vi "數位積分適應性控制_輸入權重係數_隔振(實際控制).vi"() -> ()   [LabVIEW 2010]
uses:
  <vilib>/DAQmx/read.llb/DAQmx Read (Analog DBL 1Chan 1Samp).vi
  <vilib>/DAQmx/write.llb/DAQmx Write (Analog DBL 1Chan 1Samp).vi
  <vilib>/DAQmx/create/channels.llb/DAQmx Create Channel (AI-Voltage-Basic).vi
  <vilib>/DAQmx/configure/timing.llb/DAQmx Timing (Sample Clock).vi
  <vilib>/DAQmx/create/channels.llb/DAQmx Create Channel (AO-Voltage-Basic).vi
  <vilib>/daqmx/miscellaneous.llb/DAQmx Fill In Error Info.vi
  <vilib>/measure/maspectr.llb/FFT Spectrum (Mag-Phase) for 1 Chan.vi
  <vilib>/measure/NI_MAPro.lvlib
panel:
  in  "DA輸出DC濾除":dbl
  out "積分":dbl(graph)
  in  "I增益":dbl=1.0
  in  "averaging parameters":T1={"averaging mode"=enum."No averaging", "weighting mode"=enum."Exponential", "number of averages"=10} {"number of averages" min=1}
  out "magnitude":cluster{"f0":dbl, "df":dbl, "magnitude":dbl[]} {"magnitude" format="%.2p"; "f0" format="%0.2p"; "df" format="%0.2p"}
  out "Waveform Graph":cluster{"f0":dbl, "df":dbl, "magnitude":dbl[]}(graph)
  in  "DAQ input":tag
  in  "DAQ output":tag
  in  "平均數":i32=1
  in  "ÂoDC«á©ñ¤j":dbl=1.0
  in  "Kp":dbl
  out "當下誤差":dbl=0.1 format="%#_13g"
  out "模擬輸入x(t)":dbl[][](graph)
  out "理想與FIR輸出":dbl[][](graph)
  out "message":string=" INSTRUCTIONS:\r\rNormal Use:  When using subVIs that incorporate the error in/error out (or error I/O) structure, place this handler where you want to inform the user of an error, typically at the end of the I/O data path, as the last action of the program.  If the error in error? is ERROR, the handler creates a message describing the error and its source.  If the type of dialog = 1 (default), the message is displayed to the user, who can only acknowedge it.  If the type = 2, the user can acknowledge the message or abort execution; aborting a program with active I/O is not recommended.  If the type = 0, no message is displayed; this is used to process the error programmatically, and the error out cluster elements are wired to individual terminals for that reason.  \r\rOther Use:\n\r\nlocal testing.  To test the error code of a subVI or function that does not have the error I/O structure, you can wire its error code and a source string to the local error code and error source inputs.  If error in error? indicates no error and error code is not equal to 0, the local code and source are substituted for the error in values, and error? is set TRUE (ERROR)."
  out "誤差":dbl(graph)
  out "while平均運行時間":dbl
  out "收斂time":dbl
  out "各頻率誤差已達標準":bool
  in  "各頻率誤差低於多少亮燈":dbl=0.1 format="%#_13g"
  in  "order":i32=100
  in  "取樣頻率":dbl=1000.0 min=1.0 max=1000.0 step=1.0
  in  "stop":bool
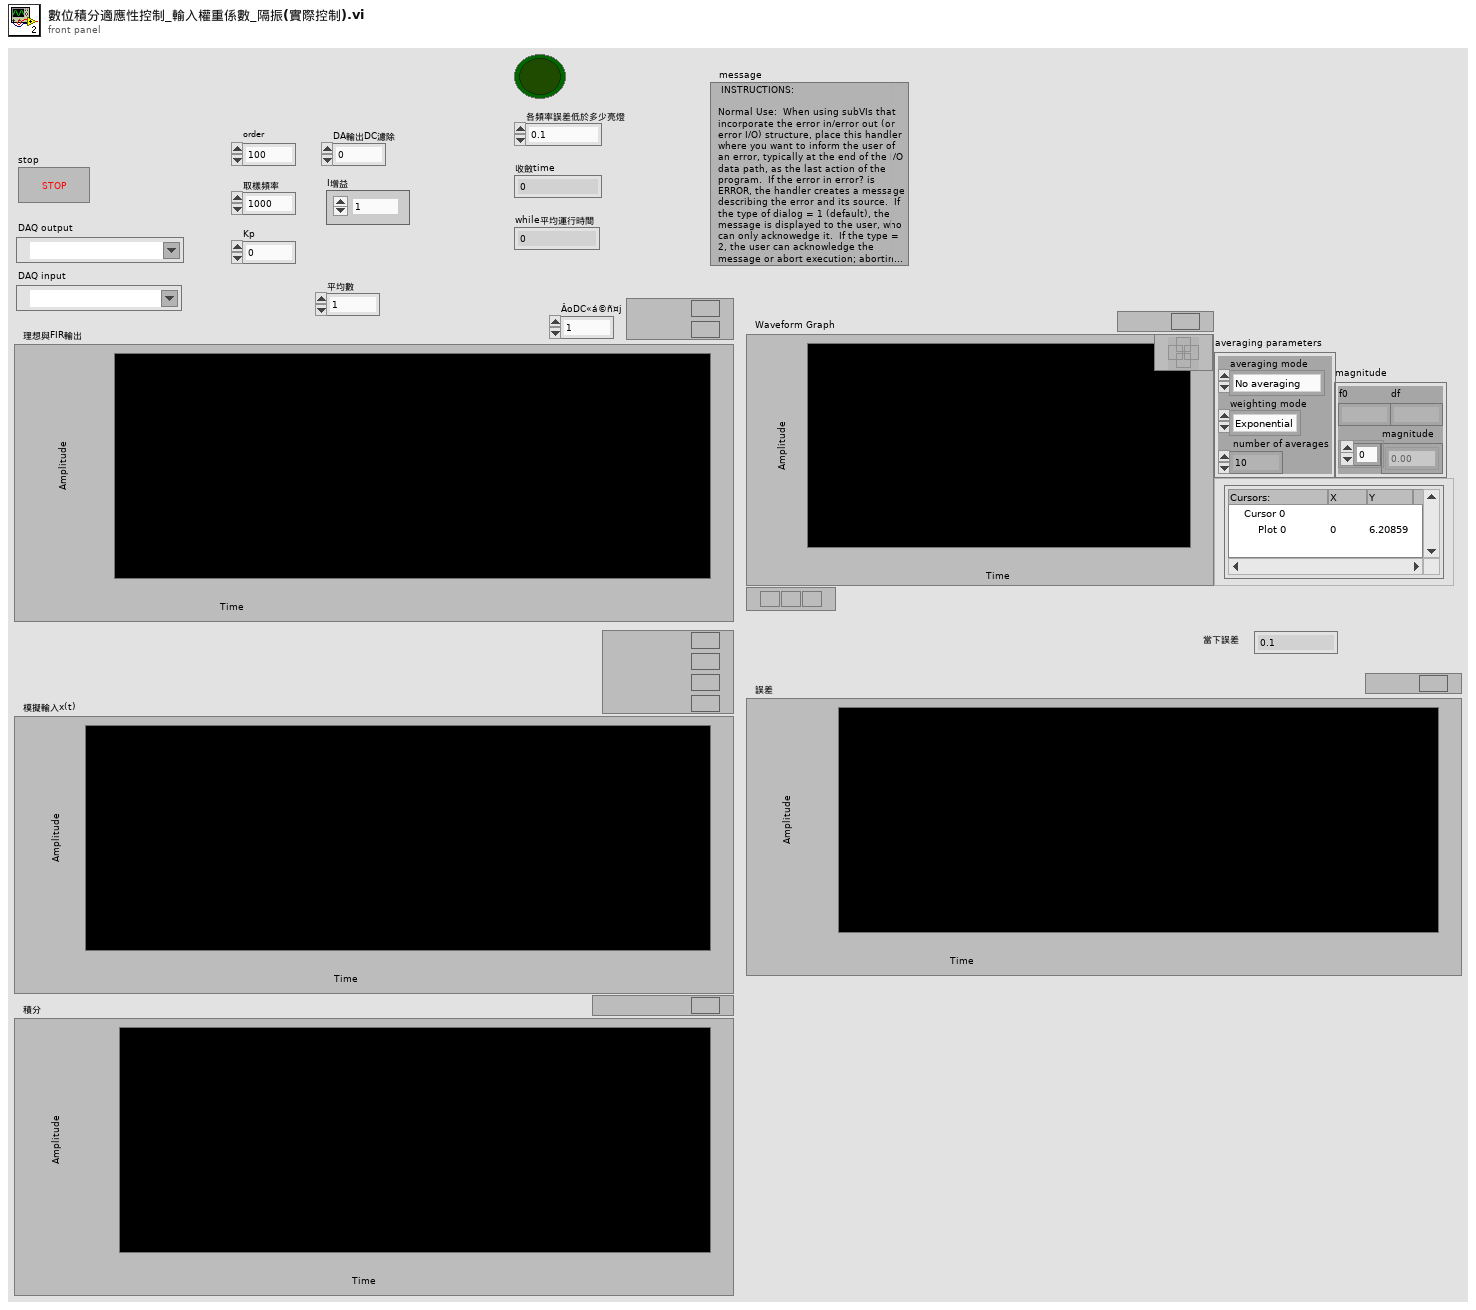
[diagram p1: front panel]
types:
  T1 = cluster{"averaging mode":enum16{"No averaging", "Vector averaging", "RMS averaging", "Peak hold"}, "weighting mode":enum16{"Linear", "Exponential"}, "number of averages":u32}
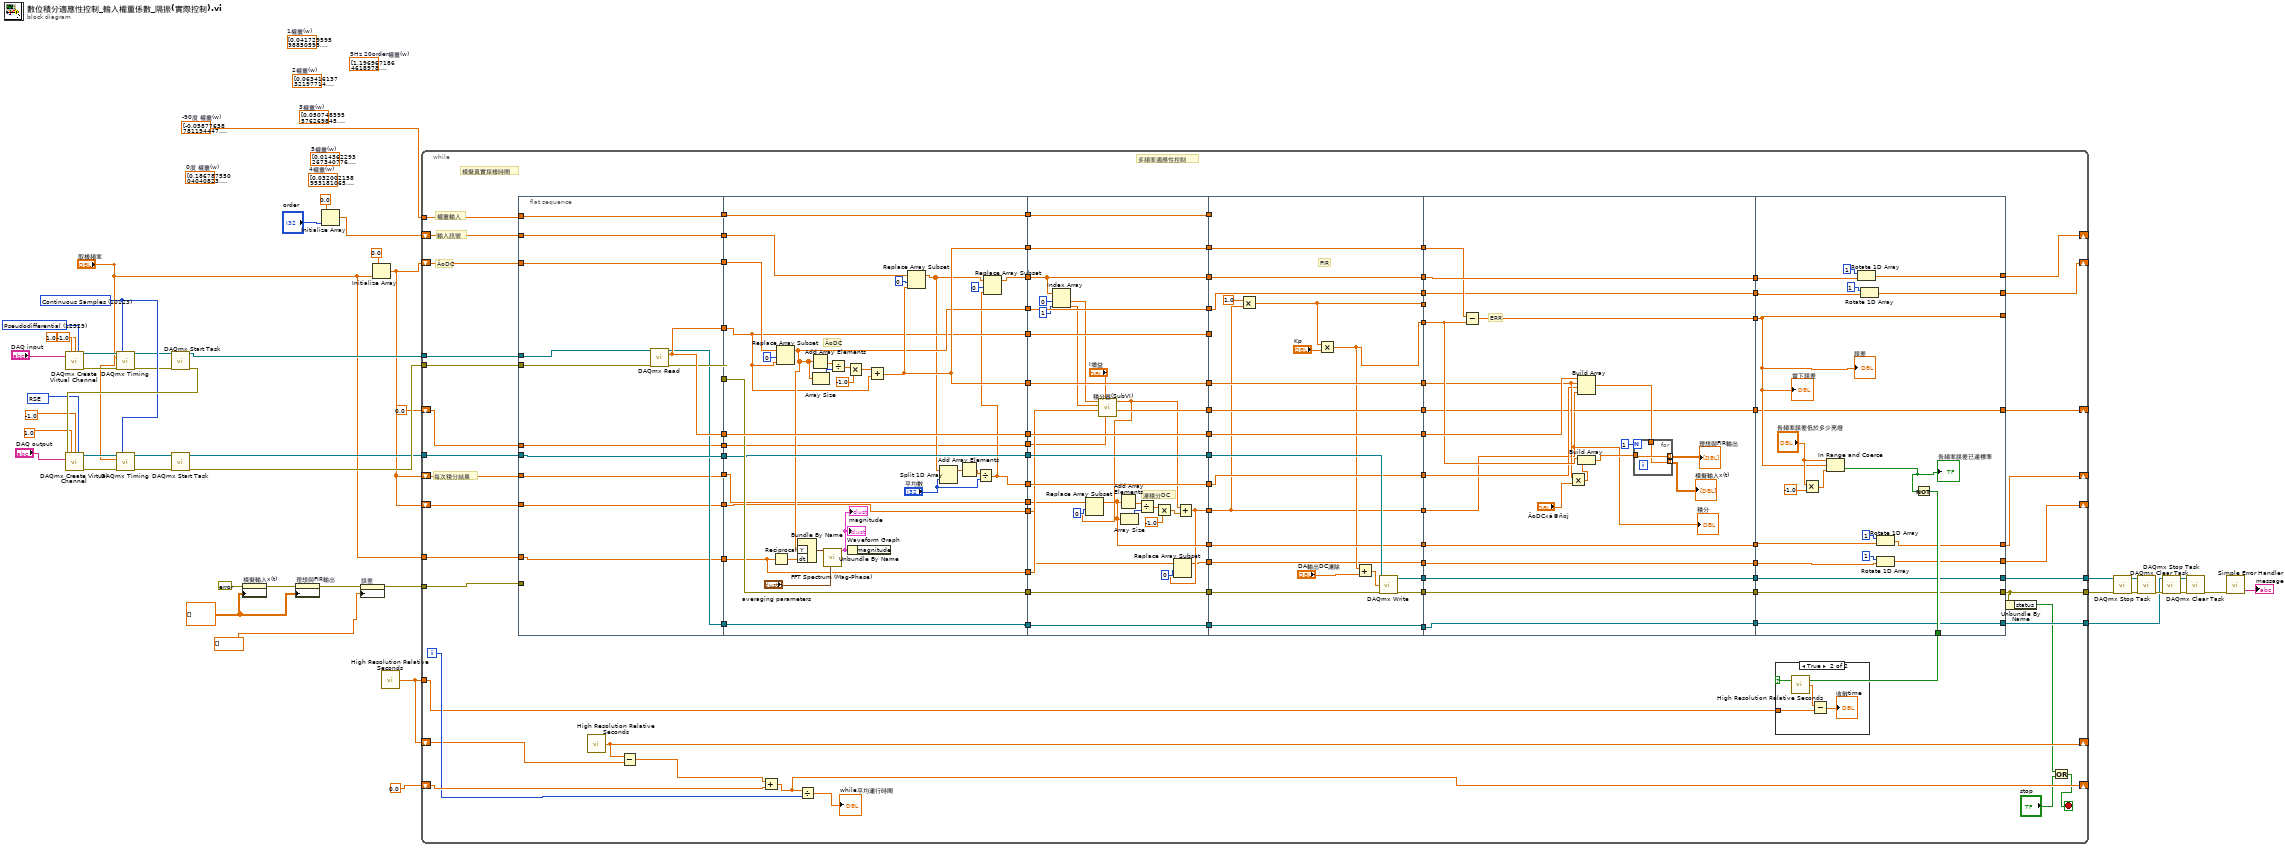
[diagram p0: block diagram]
diagram:
  (unwired) dbl[] [1.1969671864618978, 0.9836479688110593, 0.7683397307293479, 0.5547041148596448, 0.33841914564835257, 0.12405107039492207, -0.09257217575840213, -0.30706835872399124, -0.5236217829176951, -0.7376512261394793, -0.9534881580652202, -1.1673771435073645]  # 5Hz 20order權重(w)
  (unwired) dbl[] [0.04172959598850595, 0.041032000468528444, 0.040333217667049365, 0.03963360238588265, 0.03893205689600781, 0.03822950710044137, 0.03752526162041425, 0.036820019207773794, 0.03611349886737446, 0.03540561191052648, 0.03469552473426457, 0.0339838941268913, 0.03327051237657309, 0.03255595284486474, 0.031839823725201506, 0.03112222992536054, 0.030402869704382152, 0.029681974372377747, 0.02896038916329569, 0.02823777554389203, 0.027514172218931345, 0.026789142915512532, 0.026062835909340894, 0.025335140782112305, 0.0246063929857642, 0.0238764912383573, 0.023144908178161352, 0.022411287738477562, 0.021676068818243868, 0.020939160662649045, 0.020201152434326186, 0.019461448759074126, 0.018720614589735427, 0.017977930182099557, 0.017234725633515236, 0.016490584286721673, 0.01574616922561371, 0.015000724778555387, 0.014255051294173798, 0.013507854465542396, 0.012760442794157674, 0.01201235390633865, 0.011264924754863731, 0.010516019014728371, 0.009767013836059027, 0.009016973363734176, 0.008267381865193765, 0.007517321284663236, 0.006767505174674699, 0.006017229643389848, 0.005267192614920231, 0.004517461974244641, 0.003768561212744832, 0.0030200228117672986, 0.0022719427566014736, 0.0015237938881411776, 0.000776028895793179, 2.8406698505853e-05, -0.0007189560856639669, -0.001466289375680223, -0.0022141752119242833, -0.00296223837493176, -0.0037105231609250904, -0.0044587188414679894, -0.005206880706007413, -0.005954925695853661, -0.006703250220456672, -0.007451258574261906, -0.008198646895597017, -0.00894538586732751, -0.009691718602987901, -0.010437630253585128, -0.011183561844381799, -0.011928876798359233, -0.01267392362649141, -0.013418115373255173, -0.014162730174135814, -0.014907011099846127, -0.015651466362883223, -0.016395255132347217]  # 1權重(w)
  (unwired) dbl[] [0.06341613732197714, 0.06217259987768136, 0.06091889839827501, 0.059657027975942634, 0.05838513130060538, 0.057105429036780835, 0.05581630468491692, 0.05451958671274844, 0.05321400052382132, 0.05190095795462464, 0.0505792924357668, 0.04925037382622508, 0.04791324745250905, 0.04656910885733873, 0.04521739323286119, 0.04385903504088003, 0.04249355654291914, 0.04112170973577467, 0.03974339566502147, 0.038359057729198356, 0.036968896626547745, 0.035573135462967795, 0.03417200396401437, 0.032765454453403224, 0.031353955225041454, 0.029937447677999423, 0.028516571076552054, 0.02709070831884093, 0.025660911022225244, 0.02422642146811649, 0.022788545963313027, 0.02134634309175934, 0.019901312467275358, 0.01845212060283792, 0.017000713743516246, 0.015545555821830101, 0.014088891066951667, 0.01262886119459867, 0.011167931860344331, 0.009704011220608925, 0.00823993912579386, 0.006773494080066802, 0.005307599202569423, 0.0038399997075308293, 0.002373301534065933, 0.0009056073754654906, -0.0005608198104424876, -0.0020274908023066064, -0.00349257184291716, -0.00495735756770476, -0.006420298603255164, -0.007882348498007218, -0.009342158197245886, -0.010800492054227515, -0.012256318746365426, -0.013710262151131126, -0.015161545855611632, -0.016610444212633524, -0.018056301789600413, -0.019499278202438776, -0.02093899944369821, -0.0223752878332073, -0.023808034087866817, -0.025236799410333622, -0.02666156671827483, -0.028081824430815434, -0.029497837036270607, -0.030908780471520174, -0.03231490792980266, -0.033715380043063486, -0.035110769547232086, -0.03650002949596311, -0.037884088770354214, -0.039261583529015806, -0.0406335817714926, -0.0419984699060945, -0.04335769969455247, -0.044709340565506045, -0.046054929901912504, -0.04739266586653418]  # 2權重(w)
  (unwired) dbl[] [0.050748595576269845, 0.04976296352033009, 0.04875982009079402, 0.047739876462819145, 0.046703040375167114, 0.045650133074210314, 0.04458114196253071, 0.043496793229900375, 0.04239715058244961, 0.041282877646379335, 0.04015408828621526, 0.0390114226735173, 0.037855066530000724, 0.03668563212746908, 0.035503373306480325, 0.03430887198349752, 0.03310241847891101, 0.03188456159293401, 0.0306556647988646, 0.029416231366791036, 0.028166666899342822, 0.02690742906046231, 0.02563897199169044, 0.024361700257702942, 0.023076128947505922, 0.021782639152128802, 0.020481775548324012, 0.01917386761510714, 0.017859527855722725, 0.01653903984113062, 0.0152130943393199, 0.013881909276752508, 0.012546252987204293, 0.011206249418488282, 0.009862751954706962, 0.008515824389261194, 0.0071664350548475515, 0.005814557083491869, 0.004461193842393036, 0.0031062458409534983, 0.0017508549797988996, 0.00039490673524854455, -0.0009604508081786534, -0.00231532314495768, -0.0036687042224219026, -0.005020621356114889, -0.006370100664414814, -0.007717078846704026, -0.009060706958838661, -0.010400857399114933, -0.011736764664452096, -0.013068202046663332, -0.014394482563247228, -0.015715318779835633, -0.017030103015260322, -0.018338500437555277, -0.019639965699944875, -0.02093411125155473, -0.022220425174011453, -0.023498500316211767, -0.02476788628580389, -0.026028118442952625, -0.027278791828652713, -0.028519397215787497, -0.02974957386421309, -0.030968771963779416, -0.03217669828069134, -0.03337276891488156, -0.03455672003560269, -0.03572794343441583, -0.03688624362071261, -0.03803098771018863, -0.03916204565148949, -0.040278760392357484, -0.04138104888125941, -0.04246819906988395, -0.04354020353707057, -0.044596264993009734, -0.04563644214557537, -0.04666003862461791]  # 3權重(w)
  (unwired) dbl[] [0.032002158953181065, 0.03127382782707821, 0.030526170728283758, 0.029759763274351574, 0.028974940151298634, 0.028172378359730542, 0.027352456089560346, 0.026515818667865988, 0.025662886279247437, 0.024794305076083024, 0.023910519758936682, 0.02301218583560877, 0.02209978347650994, 0.021173970069008865, 0.020235260678732485, 0.019284323422338375, 0.018321690205268765, 0.017348029489250138, 0.016363905805265377, 0.015369992436563043, 0.014366868017920408, 0.013355206162749383, 0.012335601950499554, 0.011308724669250866, 0.010275192231125899, 0.009235674439598471, 0.008190803514180603, 0.007141236482790735, 0.0060876291688448, 0.005030624411114561, 0.003970920999492173, 0.00290914229363768, 0.0018460084806794317, 0.0007821062594628047, -0.0002817977090353781, -0.0013451554114184553, -0.0024071324122346663, -0.0034672373752764407, -0.004524596908236169, -0.005578769187484147, -0.006628807944435608, -0.007674293764050601, -0.00871429127788735, -0.009748368669830114, -0.010775668901956829, -0.01179573002527658, -0.01280774449609574, -0.013811208806555973, -0.014805384765904395, -0.015789748218182048, -0.016763619606387455, -0.017726453762181474, -0.018677602391468765, -0.019616511384402242, -0.02054258465159873, -0.021455266160387752, -0.022353998874567755, -0.023238226548113566, -0.02410741351803644, -0.024961012340757562, -0.02579852094447031, -0.026619400014715532, -0.02742317752943987, -0.02820932418227676, -0.02897739076641073, -0.029726858427100978, -0.030457326187173502, -0.031168284206444605, -0.031859363152719686, -0.03253006838100269, -0.033180076868829615, -0.03380889649251497, -0.034416256941201144, -0.035001681449908936, -0.035564938807506684, -0.03610554595895217, -0.0366233294436314, -0.037117764767889326, -0.037588745519972454, -0.038035863428471775]  # 4權重(w)
  (unwired) dbl[] [0.014362293267340776, 0.013689395410719023, 0.01300309315294107, 0.012304038900019095, 0.011592878877058704, 0.010870379633601756, 0.010137194353703931, 0.009394105249200462, 0.00864177649435847, 0.00788101488995614, 0.007112496730501849, 0.006337046071486811, 0.005555358538019961, 0.004768287479898683, 0.003976539913125064, 0.003180982341088728, 0.002382325980315668, 0.0015814283651622496, 0.0007790146642582781, -2.4054313914244825e-05, -0.000827057668575488, -0.0016291403226613053, -0.0024295741343070406, -0.0032275334039682992, -0.004022269261344749, -0.0048129686579806655, -0.00559888187871097, -0.006379225608899076, -0.007153234872105012, -0.007920156980446848, -0.008679209089775429, -0.009429667974273952, -0.010170745252987659, -0.010901778533758563, -0.011621962330653905, -0.012330695089693547, -0.013027139313185958, -0.013710766073403635, -0.014380735105048734, -0.015036588270713053, -0.015677454578137223, -0.016302915317597706, -0.016912126659931886, -0.0175047023962845, -0.018079862708683603, -0.018637231671910448, -0.01917608031986532, -0.01969603812834782, -0.02019644130835423, -0.020676932921196416, -0.021136920452136273, -0.021576054554505567, -0.02199380752971395, -0.022389849161288427, -0.0227637296729414, -0.023115144960455324, -0.023443713070951836, -0.02374914535548648, -0.024031129622389645, -0.024289402699926976, -0.024523719881827128, -0.024733831852911652, -0.024919569057548743, -0.02508070675145801, -0.0252171314190388, -0.02532864160374426, -0.025415208320913384, -0.0254766588913466, -0.025513034867214377, -0.02552418292972814, -0.02551021895948809, -0.025471025546434167, -0.025406810325759623, -0.02531747583831068, -0.025203309274158328, -0.025064224461733845, -0.024900580975780743, -0.02471227517816193, -0.024499764141358703, -0.024263080705131754]  # 5權重(w)
  (unwired) dbl[] [0.18678755004040823, 0.17882619748458314, 0.170712296455689, 0.16245257152505876, 0.15405454867553942, 0.14552523682324905, 0.13687159530574372, 0.12810196462388707, 0.11922362147035999, 0.11024393073088701, 0.10117036364485271, 0.09201149209306575, 0.08277436332911685, 0.07346739409850038, 0.06409841525561331, 0.05467582605915196, 0.04520705780003369, 0.03570079633951639, 0.02616517534237316, 0.016608099867348597, 0.007037550190427917, -0.002537488532805972, -0.012109386514070251, -0.021670078710663815, -0.031211136355664814, -0.04072404103843337, -0.050201506295751895, -0.059634697247062, -0.06901578876295462, -0.07833678686397391, -0.0875896165139027, -0.09676628530049372, -0.1058592127633476, -0.11486053312230449, -0.12376230508663352, -0.13255713450591536, -0.1412373426283469, -0.1497958727547784, -0.15822474190263155, -0.1665175154150831, -0.1746667650614144, -0.18266518234592094, -0.19050584543113128, -0.1981828435843626, -0.2056888768059049, -0.2130178209590218, -0.22016340348000582, -0.22711953829571419, -0.233880164162633, -0.24043951812605066, -0.2467920977101983, -0.25293205077048525, -0.2588545397521522, -0.2645544847915611, -0.27002654535583903, -0.2752661953902621, -0.28026944958627037, -0.28503187047512585, -0.28954881763286344, -0.29381678537090966, -0.29783232335913956, -0.30159129471393037, -0.3050912331475972, -0.30832924646728915, -0.3113020963534453, -0.3140069410480377, -0.31644199138653817, -0.3186047046785827, -0.3204935982376899, -0.32210684992236727, -0.32344335057664403, -0.3245013187862961, -0.3252801022894491, -0.32577926591498596, -0.32599826290987993, -0.32593663650954463, -0.32559487153422917, -0.3249726147434439, -0.3240708551869918, -0.3228901701852509]  # 0度 權重(w)
  w4 = dbl[] [-0.05877658781194447, -0.05880165783072071, -0.058769626713902144, -0.05868052843544654, -0.05853445290663261, -0.05833154600716313, -0.05807200513047942, -0.05775609051408422, -0.05738411490100067, -0.05695643829566999, -0.05647347561480095, -0.05593570222205698, -0.05534364366063041, -0.0546978771243554, -0.05399903471184836, -0.05324779605889828, -0.052444887701321614, -0.05159109221709506, -0.050687246789522196, -0.04973422883689582, -0.04873296289280662, -0.04768442344356334, -0.046589627008202315, -0.04544963505892205, -0.044265561327572645, -0.043038556514139834, -0.041769807581880536, -0.04046054418500069, -0.03911204002747684, -0.03772560321594224, -0.0363025799259075, -0.03484435512137173, -0.033352340191170726, -0.03182797732145333, -0.030272749521124433, -0.02868816831319295, -0.027075769660101768, -0.025437116513894426, -0.02377379954828862, -0.022087426486926968, -0.020379633339138514, -0.018652081796517977, -0.01690644743242602, -0.01514441726000822, -0.013367701416755104, -0.01157802234878765, -0.009777114554821144, -0.007966727150988276, -0.006148619219587733, -0.00432454880331794, -0.0024962812704839394, -0.0006655945165545307, 0.0011657354252903728, 0.002995933356237631, 0.004823221823050019, 0.006645830331619849, 0.00846199503756085, 0.010269953129429738, 0.012067944536500928, 0.01385422736721719, 0.015627071128350007, 0.01738475403707428, 0.01912557209081219, 0.020847837381648134, 0.022549872651853698, 0.02423002464683928, 0.02588666747979125, 0.027518193376758496, 0.029123015099837102, 0.03069957472506095, 0.032246340970037195, 0.03376180823956406, 0.035244507411115795, 0.036693002110996215, 0.038105881963939006, 0.039481769906701984, 0.04081933200018057, 0.042117268135363845, 0.04337431575808651, 0.04458925443984995]  # -90度 權重(w)
  w31 = 10123 items=["Finite Samples"=10178, "Continuous Samples"=10123, "Hardware Timed Single Point"=12522] ("sample mode")
  w28 = 10083 items=["Default"=-1, "RSE"=10083, "Differential"=10106, "Pseudodifferential"=12529] ("output terminal configuration")
  w27 = 12529 items=["default"=-1, "RSE"=10083, "NRSE"=10078, "Differential"=10106, "Pseudodifferential"=12529] ("input terminal configuration")
  w35 = dbl[][] [] ("History Data")
  n1 = call-poly <vilib>:"DAQmx Create Virtual Channel.vi"("maximum value"=1.0, "minimum value"=-1.0, "input terminal configuration"=w27, "physical channels"="DAQ input") -> ("task out"=w19:refnum<k21>, "error out"=w22:errorcluster)  [unwired: 10 in]
  n2 = call-poly <vilib>:"DAQmx Timing.vi"("task/channels in"=w19, "sample mode"=w31, "rate"="取樣頻率", "error in"=w22) -> ("task out"=w20:refnum<k21>, "error out"=w21:errorcluster)  [unwired: 10 in]
  n3 = call <vilib>:"DAQmx Start Task.vi"("task/channels in"=w20, "error in"=w21) -> ("task out"=w18:refnum<k21>, "error out"=w34:errorcluster)  [unwired: 12 in]
  n4 = call-poly <vilib>:"DAQmx Create Virtual Channel.vi"("maximum value"=1.0, "minimum value"=-1.0, "output terminal configuration"=w28, "physical channels"="DAQ output", "error in"=w34) -> ("task out"=w26:refnum<k21>, "error out"=w23:errorcluster)  [unwired: 9 in]
  n5 = call-poly <vilib>:"DAQmx Timing.vi"("task/channels in"=w26, "sample mode"=w31, "rate"="取樣頻率", "error in"=w23) -> ("task out"=w25:refnum<k21>, "error out"=w24:errorcluster)  [unwired: 10 in]
  n6 = call <vilib>:"DAQmx Start Task.vi"("task/channels in"=w25, "error in"=w24) -> ("task out"=w16:refnum<k21>, "error out"=w17:errorcluster)  [unwired: 12 in]
  n7 = property on="模擬輸入x(t)" class="WFChart (strict)"(error in=errorcluster {"status"=FALSE, "code"=0, "source"=""} ("error constant"), "History Data"=w35) -> (error out=w41:errorcluster)  [unwired: 1 in, 1 out]
  n8 = property on="理想與FIR輸出" class="WFChart (strict)"(error in=w41, "History Data"=w35) -> (error out=w42:errorcluster)  [unwired: 1 in, 1 out]
  n9 = Initialize Array(0.0 ("element"), "order") -> (w37:dbl[])
  n10 = property on="誤差" class="WFChart (strict)"(error in=w42, "History Data"=dbl[] []) -> (error out=w44:errorcluster)  [unwired: 1 in, 1 out]
  n11 = Initialize Array(0.0 ("element"), "取樣頻率") -> (w1:dbl[])
  n12 = call <vilib>:"High Resolution Relative Seconds.vi"() -> ("relative seconds"=w46:dbl)
  n13 = while {
    shift-right: [w123] -> _
    shift-left: w37 -> [w143]
    tunnel: w46 -> [w129]
    shift-right: [w130] -> _
    shift-left: w46 -> [w128]
    shift-right: [w131] -> _
    shift-left: 0.0 -> [w133]
    tunnel: w44 -> [w126]
    tunnel: w4 -> [w140]
    shift-right: [w117] -> _
    shift-left: w1 -> [w119]
    tunnel: w18 -> [w113]
    tunnel: w17 -> [w112]
    tunnel: w16 -> [w111]
    tunnel: [w107] -> w10
    tunnel: [w98] -> w9
    tunnel: [w101] -> w8
    tunnel: "取樣頻率" -> [w95]
    shift-right: [w67] -> _
    shift-left: 0.0 ("element") -> [w65]
    shift-right: [w55] -> _
    shift-left: w1 -> [w62]
    shift-right: [w48] -> _
    shift-left: w1 -> [w53]
    i -> [w132]
    stop <- w100 stop-if-true
    # "每次積分結果"
    # "權重輸入"
    # "輸入訊號"
    # "ÂoDC"
    # "模擬真實採樣時間"
    # "多頻率適應性控制"
    n14 = flat-sequence {
      tunnel: [w160] -> w144
      tunnel: w143 -> [w160]
      tunnel: [w155] -> w142
      tunnel: [w159] -> w141
      tunnel: w140 -> [w159]
      tunnel: w126 -> [_]
      tunnel: [w155] -> w124
      tunnel: [w154] -> w122
      tunnel: w119 -> [w158]
      tunnel: [w158] -> w118
      tunnel: w113 -> [w157]
      tunnel: w112 -> [w156]
      tunnel: w111 -> [w153]
      tunnel: [w153] -> w110
      tunnel: [w152] -> w104
      tunnel: w95 -> [w151]
      tunnel: [w151] -> w94
      tunnel: [w150] -> w66
      tunnel: w65 -> [w150]
      tunnel: [w149] -> w63
      tunnel: w62 -> [w149]
      tunnel: [w148] -> w54
      tunnel: w53 -> [w148]
      tunnel: w144 -> [w191]
      tunnel: w142 -> [w169]
      tunnel: [w167] -> w93
      tunnel: [w192] -> w91
      tunnel: w141 -> [w192]
      tunnel: [w188] -> w89
      tunnel: [w190] -> w87
      tunnel: w124 -> [w190]
      tunnel: w122 -> [w188]
      tunnel: [w180] -> w85
      tunnel: w118 -> [w186]
      tunnel: [w172] -> w83
      tunnel: [w180] -> w81
      tunnel: [w164] -> w79
      tunnel: [w176] -> w77
      tunnel: w110 -> [w176]
      tunnel: [w175] -> w75
      tunnel: w104 -> [w175]
      tunnel: [w169] -> w73
      tunnel: w94 -> [w165]
      tunnel: [w165] -> w71
      tunnel: w66 -> [w163]
      tunnel: [w163] -> w64
      tunnel: w63 -> [w162]
      tunnel: [w162] -> w61
      tunnel: w54 -> [w161]
      tunnel: [w161] -> w52
      tunnel: w93 -> [w212]
      tunnel: [w212] -> w92
      tunnel: w91 -> [w224]
      tunnel: [w224] -> w90
      tunnel: w89 -> [w223]
      tunnel: [w223] -> w88
      tunnel: w87 -> [w222]
      tunnel: [w222] -> w86
      tunnel: w85 -> [w221]
      tunnel: [w221] -> w84
      tunnel: w83 -> [w220]
      tunnel: [w220] -> w82
      tunnel: w81 -> [w219]
      tunnel: [w219] -> w80
      tunnel: w79 -> [w218]
      tunnel: [w218] -> w78
      tunnel: w77 -> [w217]
      tunnel: [w217] -> w76
      tunnel: w75 -> [w216]
      tunnel: [w216] -> w74
      tunnel: w73 -> [w215]
      tunnel: [w215] -> w72
      tunnel: w71 -> [w214]
      tunnel: [w207] -> w69
      tunnel: w64 -> [w206]
      tunnel: w61 -> [w200]
      tunnel: [w194] -> w60
      tunnel: [w198] -> w58
      tunnel: w52 -> [w195]
      tunnel: [w193] -> w50
      tunnel: w92 -> [w234]
      tunnel: w90 -> [_]
      tunnel: [w226] -> w139
      tunnel: [w234] -> w138
      tunnel: w88 -> [w239]
      tunnel: [w245] -> w125
      tunnel: w86 -> [w245]
      tunnel: [w243] -> w121
      tunnel: w84 -> [w243]
      tunnel: [w231] -> w120
      tunnel: [w241] -> w115
      tunnel: w82 -> [w241]
      tunnel: w80 -> [w242]
      tunnel: [w242] -> w114
      tunnel: w78 -> [w235]
      tunnel: w76 -> [w240]
      tunnel: [w238] -> w108
      tunnel: [w237] -> w106
      tunnel: w74 -> [w236]
      tunnel: [w236] -> w103
      tunnel: [w235] -> w96
      tunnel: w72 -> [_]
      tunnel: [w233] -> w70
      tunnel: w69 -> [w233]
      tunnel: w60 -> [w227]
      tunnel: [w227] -> w59
      tunnel: w58 -> [w232]
      tunnel: [w232] -> w56
      tunnel: [w228] -> w51
      tunnel: w50 -> [w228]
      tunnel: w139 -> [_]
      tunnel: w138 -> [w265]
      tunnel: [w265] -> w137
      tunnel: [w263] -> w136
      tunnel: w125 -> [w261]
      tunnel: w121 -> [w262]
      tunnel: w120 -> [w259]
      tunnel: [w251] -> w116
      tunnel: w115 -> [w251]
      tunnel: w114 -> [w258]
      tunnel: [w255] -> w109
      tunnel: w108 -> [w255]
      tunnel: w106 -> [w254]
      tunnel: [w254] -> w105
      tunnel: w103 -> [w253]
      tunnel: [w253] -> w102
      tunnel: w96 -> [w252]
      tunnel: w70 -> [w250]
      tunnel: [w250] -> w68
      tunnel: w59 -> [w247]
      tunnel: [w248] -> w57
      tunnel: w56 -> [w248]
      tunnel: w51 -> [w246]
      tunnel: [w246] -> w49
      tunnel: w137 -> [w285]
      tunnel: [w291] -> w123
      tunnel: w136 -> [w283]
      tunnel: [w287] -> w127
      tunnel: [w283] -> _
      tunnel: [w281] -> w117
      tunnel: w116 -> [w280]
      tunnel: w109 -> [w279]
      tunnel: [w279] -> w107
      tunnel: [w278] -> w98
      tunnel: w105 -> [w278]
      tunnel: w102 -> [w277]
      tunnel: [w277] -> w101
      tunnel: w68 -> [w276]
      tunnel: [w276] -> w67
      tunnel: w57 -> [w274]
      tunnel: [w273] -> w55
      tunnel: w49 -> [w271]
      tunnel: [w270] -> w48
      frame #0 {
        n15 = call-poly <vilib>:"DAQmx Read.vi"("task/channels in"=w157, "error in"=w156) -> ("task out"=w152:refnum<k21>, "data"=w155:dbl, "error out"=w154:errorcluster)  [unwired: 11 in]
      }
      frame #1 {
        # "ÂoDC"
        n16 = Reciprocal(x=w165) -> (1/x=w171:dbl)
        n17 = Replace Array Subset(array=w186, new element=w169, index=0) -> (w172:dbl[])
        n18 = Bundle By Name("Y"=w172, "dt"=w171) -> (w174:waveform(dbl))  [unwired: 1 in]
        n19 = Add Array Elements(numeric array=w172) -> (sum=w185:dbl)
        n20 = Array Size(array=w172) -> (size(s)=w184:i32)
        n21 = call-poly <vilib>:"FFT Spectrum (Mag-Phase).vi"("averaging parameters"="averaging parameters", "time signal"=w174) -> ("magnitude"=w173:cluster{"f0":dbl, "df":dbl, "magnitude":dbl[]})  [unwired: 5 in, 4 out]
        "Waveform Graph" <- w173
        "magnitude" <- w173
        n22 = Divide(x=w185, y=w184) -> (x/y=w183:dbl)
        n23 = Multiply(x=w183, y=-1.0) -> (x*y=w181:dbl)
        n24 = Unbundle By Name(w173) -> ()  [unwired: 1 out]
        n25 = Add(x=w181, y=w169) -> (x+y=w180:dbl)
        n26 = Replace Array Subset(array=w191, new element=w180, index=0) -> (w168:dbl[])
        n27 = Split 1D Array(array=w168, index="平均數") -> (first subarray=w179:dbl[])  [unwired: 1 out]
        n28 = Add Array Elements(numeric array=w179) -> (sum=w178:dbl)
        n29 = Divide(x=w178, y="平均數") -> (x/y=w164:dbl)
        n30 = Replace Array Subset(array=w168, new element=w164, index=0) -> (w167:dbl[])
      }
      frame #2 {
        # "濾積分DC"
        n31 = Index Array(array=w212, index #1=0 ("index"), index #2=1 ("index")) -> (element #1=w209:dbl, element #2=w208:dbl)
        n32 = call "積分器(SubVI).vi"("輸入累加ERR回朔"=w206, "I增益"="I增益", "samples (Hz)"=w214, "前一個ERR"=w208, "當下ERR"=w209) -> ("輸出累加ERR回朔"=w207:dbl, "積分修正量"=w199:dbl)  [unwired: 5 in]
        n33 = Replace Array Subset(array=w200, new element=w199, index=0) -> (w198:dbl[])
        n34 = Add Array Elements(numeric array=w198) -> (sum=w202:dbl)
        n35 = Array Size(array=w198) -> (size(s)=w203:i32)
        n36 = Divide(x=w202, y=w203) -> (x/y=w204:dbl)
        n37 = Multiply(x=w204, y=-1.0) -> (x*y=w197:dbl)
        n38 = Add(x=w199, y=w197) -> (x+y=w194:dbl)
        n39 = Replace Array Subset(array=w195, new element=w194, index=0) -> (w193:dbl[])
      }
      frame #3 {
        # "FIR"
        n40 = Multiply(x=1.0, y=w227) -> (x*y=w226:dbl)
        n41 = Multiply(x=w226, y="Kp") -> (x*y=w231:dbl)
        n42 = Add(x=w231, y="DA輸出DC濾除") -> (x+y=w229:dbl)
        n43 = call-poly <vilib>:"DAQmx Write.vi"("task/channels in"=w240, "data"=w229, "error in"=w239) -> ("task out"=w238:refnum<k21>, "error out"=w237:errorcluster)  [unwired: 10 in, 1 out]
      }
      frame #4 {
        # "ERR"
        n44 = Subtract(x=w262, y=w259) -> (x-y=w263:dbl)
        n45 = Multiply(x=w258, y="ÂoDC«á©ñ¤j") -> (x*y=w256:dbl)
        n46 = Build Array(w261, w258, w252, w247) -> (w260:dbl[])
        n47 = Build Array(w259, w256) -> (w249:dbl[])
        n48 = for {
          N: 1 -> [_]
          tunnel: [w269] -> w264 mode=indexing
          tunnel: w249 -> [w269]
          tunnel: [w268] -> w266 mode=indexing
          tunnel: w260 -> [w268]
        }
        "理想與FIR輸出" <- w264
        "模擬輸入x(t)" <- w266
        "積分" <- w247
      }
      frame #5 {
        n49 = Multiply(x="各頻率誤差低於多少亮燈", y=-1.0) -> (x*y=w288:dbl)
        n50 = In Range and Coerce(upper limit="各頻率誤差低於多少亮燈", x=w283, lower limit=w288) -> (In Range?=w284:bool)  [unwired: 1 out]
        "各頻率誤差已達標準" <- w284
        n51 = Rotate 1D Array(1:w285, 2:1 ("n")) -> (0:w291:dbl[])
        n52 = Rotate 1D Array(1:w280, 2:1 ("n")) -> (0:w281:dbl[])
        n53 = Rotate 1D Array(1:w274, 2:1 ("n")) -> (0:w273:dbl[])
        n54 = Rotate 1D Array(1:w271, 2:1 ("n")) -> (0:w270:dbl[])
        n55 = Not(x=w284) -> (.not. x?=w287:bool)
        "誤差" <- w283
        "當下誤差" <- w283
      }
    }
    n56 = call <vilib>:"High Resolution Relative Seconds.vi"() -> ("relative seconds"=w130:dbl)
    n57 = Subtract(x=w130, y=w128) -> (x-y=w135:dbl)
    n58 = Add(x=w135, y=w133) -> (x+y=w131:dbl)
    n59 = Divide(x=w131, y=w132) -> (x/y=→"while平均運行時間":dbl)
    n60 = case shown="True" w127 {
      tunnel: w129 -> [_ w145]
      frame False {
      }
      frame True {
        n61 = call <vilib>:"High Resolution Relative Seconds.vi"() -> ("relative seconds"=w147:dbl)
        n62 = Subtract(x=w147, y=w145) -> (x-y=→"收斂time":dbl)
      }
    }
    n63 = Unbundle By Name(w98) -> ("status"=w97:bool)
    n64 = Or(x=w97, y="stop") -> (x .or. y?=w100:bool)
  }
  n65 = call <vilib>:"DAQmx Stop Task.vi"("task/channels in"=w10, "error in"=w9) -> ("task out"=w11:refnum<k21>, "error out"=w12:errorcluster)  [unwired: 12 in]
  n66 = call <vilib>:"DAQmx Clear Task.vi"("task in"=w11, "error in"=w12) -> ("error out"=w15:errorcluster)  [unwired: 13 in]
  n67 = call <vilib>:"DAQmx Stop Task.vi"("task/channels in"=w8, "error in"=w15) -> ("task out"=w14:refnum<k21>, "error out"=w13:errorcluster)  [unwired: 12 in]
  n68 = call <vilib>:"DAQmx Clear Task.vi"("task in"=w14, "error in"=w13) -> ("error out"=w7:errorcluster)  [unwired: 13 in]
  n69 = call <vilib>:"Simple Error Handler.vi"("error in (no error)"=w7) -> ("message"=→"message":string)  [unwired: 4 in, 4 out]
